vi "Read Roles.vi"(8 "error in (no error)":errorcluster, 11 "PreparePenaltyAllyPlay in":refnum<class "PreparePenaltyAllyPlay.lvclass">) -> (0 "error out":errorcluster, 2 "Roles":T1, 3 "PreparePenaltyAllyPlay out":refnum<class "PreparePenaltyAllyPlay.lvclass">)   [LabVIEW 2023, in "PreparePenaltyAllyPlay.lvclass"]
uses:
  PreparePenaltyAllyPlay.lvclass
  AttackerAimGoalRole_class/AttackerAimGoalRole.lvclass
  PreparePenaltyAllyPlay.lvclass/PreparePenaltyAllyPlay.ctl
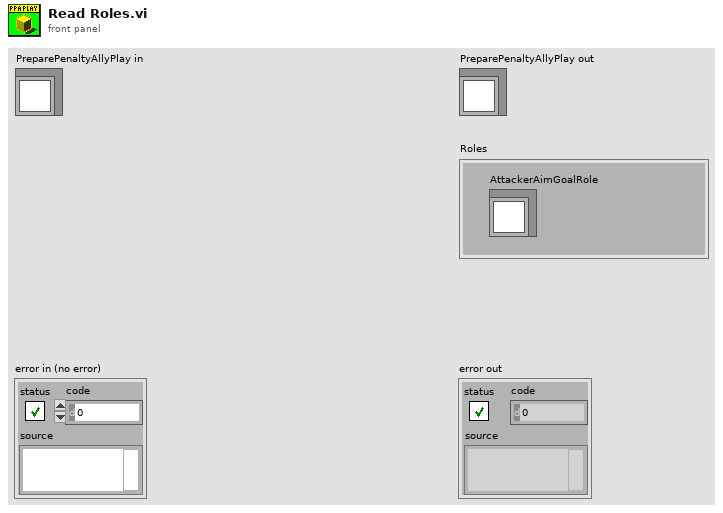
[diagram p1: front panel]
types:
  T1 = cluster{"AttackerAimGoalRole":refnum<class "AttackerAimGoalRole.lvclass">}
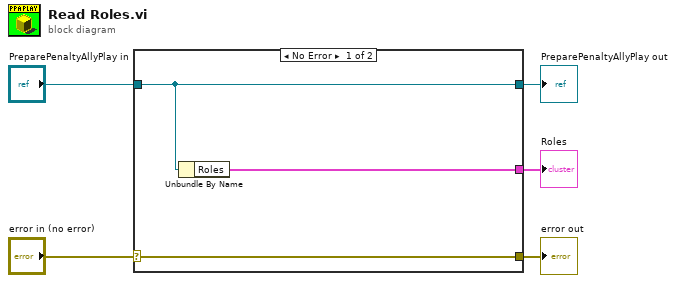
[diagram p0: block diagram]
diagram:
  n1 = case shown="No Error" "error in (no error)" {
    selector: "error in (no error)" -> [w8 w9]
    tunnel: [w8 w9] -> w4
    tunnel: [w7 w10] -> w2
    tunnel: "PreparePenaltyAllyPlay in" -> [w7 w10]
    tunnel: [w6 _] -> w1
    frame No Error {
      n2 = Unbundle By Name(w7) -> ("Roles"=w6:T1)
    }
    frame Error {
    }
  }
  "error out" <- w4
  "PreparePenaltyAllyPlay out" <- w2
  "Roles" <- w1
